vi "Aladdin 2 build.vi"() -> ()   [LabVIEW 2020]
uses:
  <vilib>/Instr/_visa.llb/VISA Configure Serial Port (Instr).vi
panel:
  in  "stop":bool
  in  "Mode":enum32{"Setup", "Run"}(tab)
  out "Min rate 2":dbl caption="Min rate" format="%#_4g"
  in  "Target Volume2":dbl caption="Target Vol (ul)"
  in  "Send 2":bool
  in  "Address2":string(combo) caption="Address"
  in  "Dia (mm)2":dbl=0.1 caption="Dia (mm)" min=0.1 max=50.0
  out "Max rate ml/min2":dbl caption="Max rate" format="%#_4g"
  in  "Direction2":string(combo)="inf" caption="Direction"
  in  "Serial Reset":bool
  in  "Target Vol":dbl caption="Target Vol (ul)"
  in  "Send":bool
  in  "Address":string(combo)
  in  "dia (mm)":dbl=0.1 caption="Dia (mm)" min=0.1 max=50.0
  out "Max rate":dbl format="%#_4g"
  in  "Direction":string(combo)="inf"
  in  "Serial Port":refnum<visa-resource-name>="COM1"
  in  "Pumps":string(combo)="1"
  in  "Set rate":dbl format="%#_4g"
  in  "Flow rate2":dbl caption="Set rate"
  out "Min rate":dbl format="%#_4g"
  in  "Units":string(combo)="mm"
  in  "Units2":string(combo)="mm" caption="Units"
  out "Dispensed 2":string caption="Dispensed"
  out "Dispensed":string
  out "Direction1":string caption="Direction"
  in  "Go 2":bool
  in  "Go 1":bool
  out "Target2":string caption="Target"
  out "Target1":string caption="Target"
  out "Direction2":string caption="Direction"
  out "Rate2":string caption="Rate"
  out "Rate1":string caption="Rate"
  in  "Reset1 2":bool
  in  "Reset1":bool
  # "Pump 1"
  # "Pump 2"
  # "Set pump Baud rate to 19200"
  # "Pump 1"
  # "Pump 2"
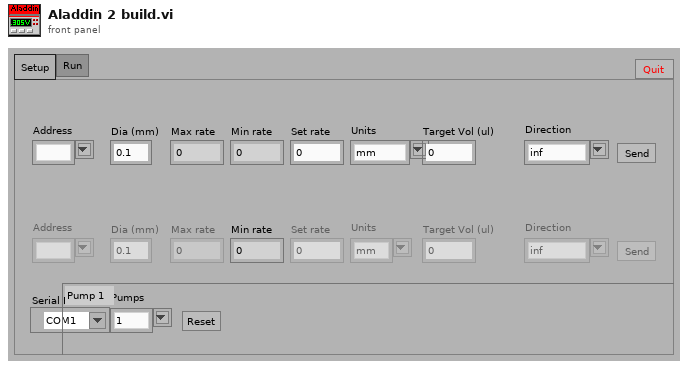
[diagram p1: front panel]
types:
  T1 = enum8{"Enabled", "Disabled", "Disabled and Grayed Out"}
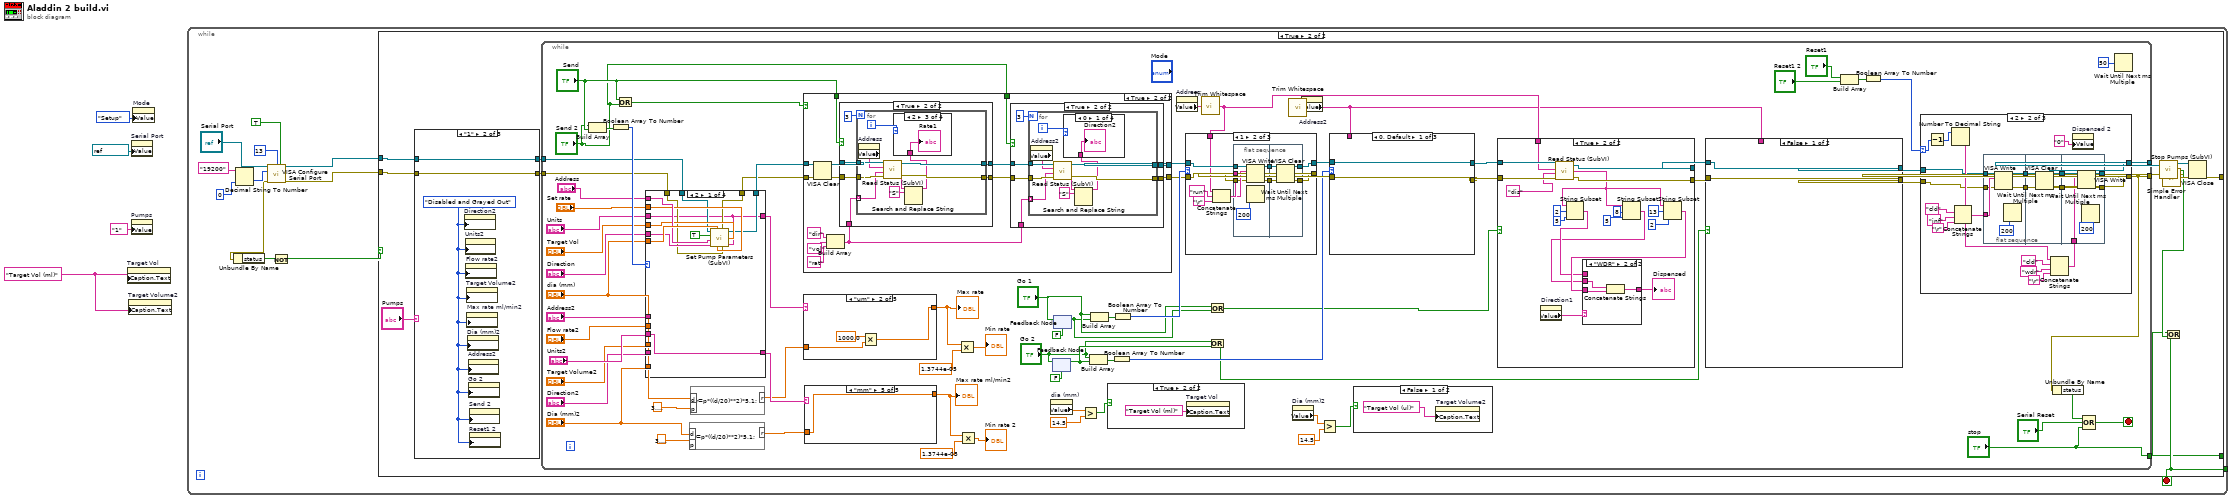
[diagram p0: block diagram]
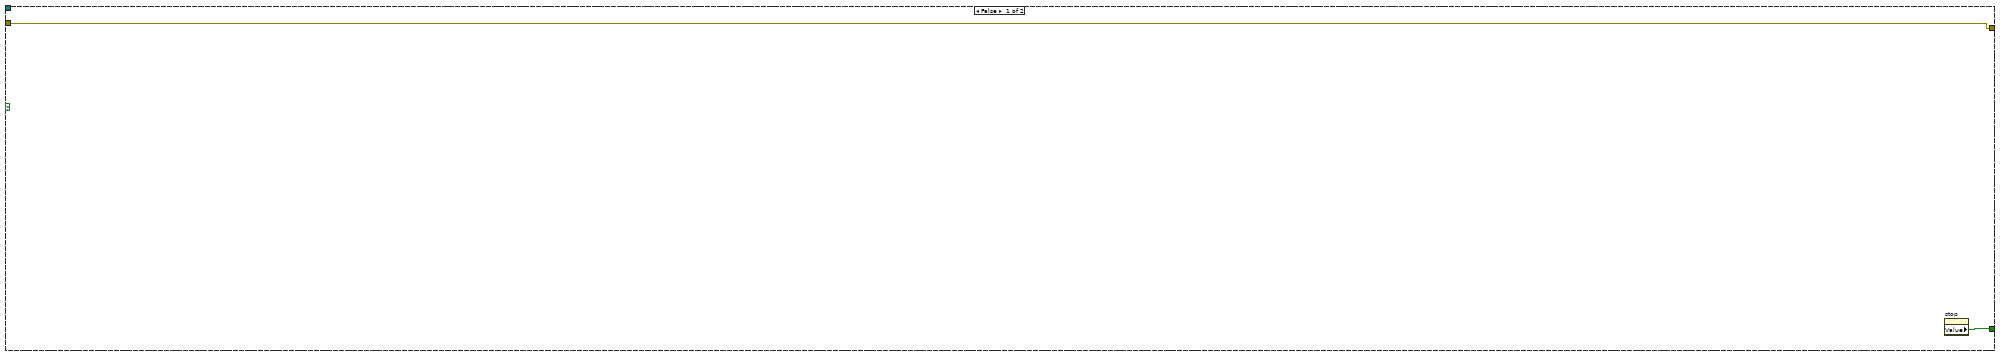
[diagram p2: hidden frame]
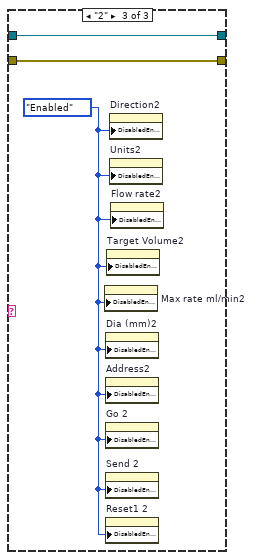
[diagram p4: hidden frame]
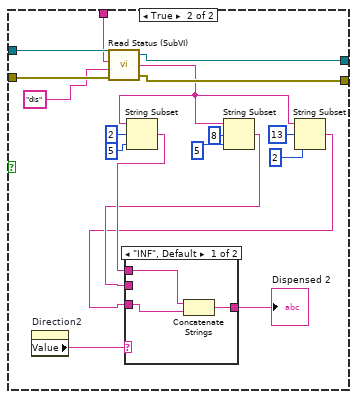
[diagram p5: hidden frame]
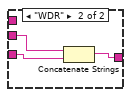
[diagram p6: hidden frame]
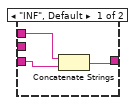
[diagram p8: hidden frame]
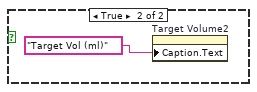
[diagram p9: hidden frame]
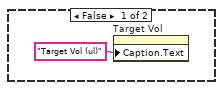
[diagram p10: hidden frame]
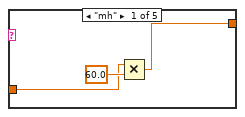
[diagram p11: hidden frame]
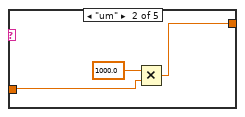
[diagram p12: hidden frame]
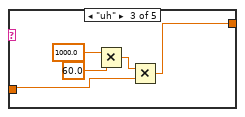
[diagram p13: hidden frame]
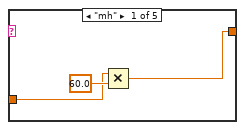
[diagram p15: hidden frame]
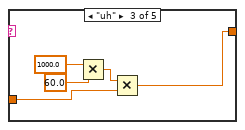
[diagram p16: hidden frame]
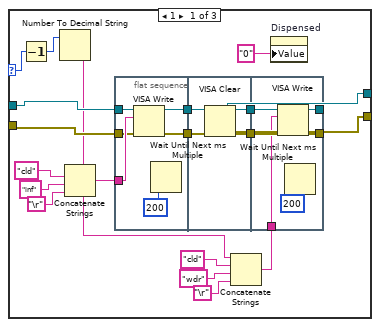
[diagram p19: hidden frame]
diagram:
  w1 = "Target Vol (ml)" ("Caption.Text")
  n1 = property on="Target Vol" class="DigNum (strict)"("Caption.Text"=w1) -> ()  [unwired: 2 in, 2 out]
  n2 = property on="Target Volume2" class="DigNum (strict)"("Caption.Text"=w1) -> ()  [unwired: 2 in, 2 out]
  n3 = property on="Serial Port" class="VISAName"("Value"=refnum<visa-resource-name> "COM1" ("Serial Port")) -> ()  [unwired: 2 in, 2 out]
  n4 = property on="Pumps" class="CmbBox"("Value"="1" ("Pumps")) -> ()  [unwired: 2 in, 2 out]
  n5 = property on="Mode" class="TabCtl (strict)"("Value"=enum32{"Setup", "Run"}."Setup" ("Mode")) -> ()  [unwired: 2 in, 2 out]
  n6 = while {
    tunnel: [w7] -> _
    stop <- w7 stop-if-true
    n7 = Decimal String To Number(string="19200" ("Baud Rate"), default (0L)=u32 0 ("default (0 I32)")) -> (number=w14:u32)  [unwired: 1 in, 1 out]
    n8 = call-poly "VISA Configure Serial Port"("VISA resource name"="Serial Port", "termination char\n(0xA = '\\n' = LF)"=u8 13 ("termination char\n(0xA = '\\n' = LF)"), "Enable Termination\nChar (T)"=TRUE ("Enable Termination\nChar (T)"), "baud rate (9600)"=w14) -> ("VISA resource name out"=w12:refnum<visa-resource-name>, "error out"=w10:errorcluster)  [unwired: 10 in]
    n9 = Unbundle By Name(w10) -> ("status"=w9:bool)
    n10 = Not(x=w9) -> (.not. x?=w8:bool)
    n11 = case shown="True" w8 {
      tunnel: w12 -> [_ w28]
      tunnel: w10 -> [w20 w27]
      tunnel: [w19 w24] -> w5
      tunnel: [w20 w21] -> w11
      frame False {
        n12 = property on="stop" class="Bool (strict)"() -> ("Value"=w19:bool)  [unwired: 2 in, 2 out]
      }
      frame True {
        n13 = case shown="\"1\"" "Pumps" {
          tunnel: w28 -> [w33 w35 w38]
          tunnel: w27 -> [w32 w34 w37]
          tunnel: [w33 w35 w38] -> w26
          tunnel: [w32 w34 w37] -> w25
          frame Default {
          }
          frame "1" {
            w36 = T1."Disabled and Grayed Out" ("Disabled")
            n14 = property on="Direction2" class="CmbBox"("DisabledEnum"=w36) -> ()  [unwired: 2 in, 2 out]
            n15 = property on="Units2" class="CmbBox"("DisabledEnum"=w36) -> ()  [unwired: 2 in, 2 out]
            n16 = property on="Flow rate2" class="DigNum (strict)"("DisabledEnum"=w36) -> ()  [unwired: 2 in, 2 out]
            n17 = property on="Target Volume2" class="DigNum (strict)"("DisabledEnum"=w36) -> ()  [unwired: 2 in, 2 out]
            n18 = property on="Max rate ml/min2" class="DigNum (strict)"("DisabledEnum"=w36) -> ()  [unwired: 2 in, 2 out]
            n19 = property on="Dia (mm)2" class="DigNum (strict)"("DisabledEnum"=w36) -> ()  [unwired: 2 in, 2 out]
            n20 = property on="Address2" class="CmbBox"("DisabledEnum"=w36) -> ()  [unwired: 2 in, 2 out]
            n21 = property on="Go 2" class="Bool (strict)"("DisabledEnum"=w36) -> ()  [unwired: 2 in, 2 out]
            n22 = property on="Send 2" class="Bool"("DisabledEnum"=w36) -> ()  [unwired: 2 in, 2 out]
            n23 = property on="Reset1 2" class="Bool"("DisabledEnum"=w36) -> ()  [unwired: 2 in, 2 out]
          }
          frame "2" {
            w39 = T1."Enabled" ("Disabled")
            n24 = property on="Max rate ml/min2" class="DigNum (strict)"("DisabledEnum"=w39) -> ()  [unwired: 2 in, 2 out]
            n25 = property on="Dia (mm)2" class="DigNum (strict)"("DisabledEnum"=w39) -> ()  [unwired: 2 in, 2 out]
            n26 = property on="Address2" class="CmbBox"("DisabledEnum"=w39) -> ()  [unwired: 2 in, 2 out]
            n27 = property on="Go 2" class="Bool (strict)"("DisabledEnum"=w39) -> ()  [unwired: 2 in, 2 out]
            n28 = property on="Send 2" class="Bool"("DisabledEnum"=w39) -> ()  [unwired: 2 in, 2 out]
            n29 = property on="Reset1 2" class="Bool"("DisabledEnum"=w39) -> ()  [unwired: 2 in, 2 out]
            n30 = property on="Target Volume2" class="DigNum (strict)"("DisabledEnum"=w39) -> ()  [unwired: 2 in, 2 out]
            n31 = property on="Direction2" class="CmbBox"("DisabledEnum"=w39) -> ()  [unwired: 2 in, 2 out]
            n32 = property on="Units2" class="CmbBox"("DisabledEnum"=w39) -> ()  [unwired: 2 in, 2 out]
            n33 = property on="Flow rate2" class="DigNum (strict)"("DisabledEnum"=w39) -> ()  [unwired: 2 in, 2 out]
          }
        }
        n34 = while {
          tunnel: w25 -> [w87]
          tunnel: w26 -> [w88]
          tunnel: ["stop"] -> w24
          tunnel: [w79] -> w30
          tunnel: [w59] -> w29
          stop <- w114 stop-if-true
          n35 = Build Array("Send 2", "Send") -> (w101:bool[])
          n36 = Boolean Array To Number(Boolean array=w101) -> (number=w100:u32)
          n37 = Or(x="Send", y="Send 2") -> (x .or. y?=w89:bool)
          n38 = case shown="2" w100 {
            tunnel: "Address" -> [w281 _ _ _]
            tunnel: "Set rate" -> [w279 _ _ _]
            tunnel: "Units" -> [w273 w286 w297 w301]
            tunnel: "Target Vol" -> [w278 _ _ _]
            tunnel: "Direction" -> [w280 _ _ _]
            tunnel: "dia (mm)" -> [w283 _ _ _]
            tunnel: "Address2" -> [_ w295 _ _]
            tunnel: "Flow rate2" -> [_ w294 _ _]
            tunnel: "Units2" -> [w272 w284 w296 w300]
            tunnel: "Target Volume2" -> [_ w293 _ _]
            tunnel: "Direction2" -> [_ w285 _ _]
            tunnel: "Dia (mm)2" -> [_ w292 _ _]
            tunnel: w88 -> [w275 w290 w298 w304]
            tunnel: w87 -> [w274 w289 w299 w303]
            tunnel: [w276 w288 w298 w304] -> w86
            tunnel: [w277 w287 w299 w303] -> w85
            tunnel: [w273 w286 w297 w301] -> w73
            tunnel: [w272 w284 w296 w300] -> w72
            frame 2 {
              n39 = call "Set Pump Parameters (SubVI).vi"("Units"=w273, "error in"=w274, "Target Volume"=w278, "Flow rate"=w279, "Direction"=w280, "Pump Add"=w281, "diameter (mm)"=w283, "Send"=TRUE, "VISA resource name in"=w275) -> ("VISA resource name out"=w276:refnum<visa-resource-name>, "error out"=w277:errorcluster)
            }
            frame 1 {
              n40 = call "Set Pump Parameters (SubVI).vi"("Units"=w284, "error in"=w289, "Target Volume"=w293, "Flow rate"=w294, "Direction"=w285, "Pump Add"=w295, "diameter (mm)"=w292, "Send"=TRUE, "VISA resource name in"=w290) -> ("VISA resource name out"=w288:refnum<visa-resource-name>, "error out"=w287:errorcluster)
            }
            frame Default {
            }
            frame 3 {
              n41 = call "Set Pump Parameters (SubVI).vi"("Send"=FALSE) -> ()  [unwired: 8 in, 2 out]
            }
          }
          n42 = formula code="r=p*((d/20)**2)*5.1;"("d"="Dia (mm)2", "p"=3.141592653589793) -> ("r"=w70:dbl)
          n43 = formula code="r=p*((d/20)**2)*5.1;"("d"="dia (mm)", "p"=3.141592653589793) -> ("r"=w71:dbl)
          n44 = case shown="True" w89 {
            tunnel: [w390 w394] -> w105
            tunnel: [w389 w393] -> w104
            tunnel: w86 -> [w390 w399]
            tunnel: w85 -> [w389 w398]
            tunnel: "Send" -> [_ w392]
            tunnel: "Send 2" -> [_ w391]
            frame False {
            }
            frame True {
              n45 = VISA Clear(VISA resource name=w399, error in (no error)=w398) -> (VISA resource name out=w401:refnum<visa-resource-name>, error out=w400:errorcluster)
              n46 = Build Array("dir", "vol", "rat") -> (w395:string[])
              n47 = case shown="True" w392 {
                tunnel: [w427 w433] -> w397
                tunnel: [w426 w432] -> w396
                tunnel: w395 -> [_ w431]
                tunnel: w401 -> [w427 w430]
                tunnel: w400 -> [w426 w429]
                frame False {
                }
                frame True {
                  n48 = for {
                    N: 3 -> [_]
                    tunnel: w430 -> [w443]
                    tunnel: w429 -> [w442]
                    tunnel: w431 -> [w441] mode=indexing
                    tunnel: [w440] -> w433
                    tunnel: [w439] -> w432
                    i -> [w435]
                    n49 = property on="Address" class="CmbBox"() -> ("Value"=w434:string)  [unwired: 2 in, 2 out]
                    n50 = call "Read Status (SubVI).vi"("error out 2"=w442, "String"=w441, "String 2"=w434, "VISA resource name out 2"=w443) -> ("error out"=w439:errorcluster, "read buffer"=w437:string, "VISA resource name out"=w440:refnum<visa-resource-name>)
                    n51 = Search and Replace String(input string=w437, search string="S") -> (result string=w436:string)  [unwired: 6 in, 3 out]
                    n52 = case shown="2" w435 {
                      tunnel: w436 -> [w444 w445 w446 _]
                      frame 0 {
                        "Direction1" <- w444
                      }
                      frame 1 {
                        "Target1" <- w445
                      }
                      frame 2 {
                        "Rate1" <- w446
                      }
                      frame Default {
                      }
                    }
                  }
                }
              }
              n53 = case shown="True" w391 {
                tunnel: [w406 w412] -> w394
                tunnel: [w405 w411] -> w393
                tunnel: w395 -> [_ w410]
                tunnel: w397 -> [w406 w409]
                tunnel: w396 -> [w405 w408]
                frame False {
                }
                frame True {
                  n54 = for {
                    N: 3 -> [_]
                    tunnel: w409 -> [w422]
                    tunnel: w408 -> [w421]
                    tunnel: w410 -> [w420] mode=indexing
                    tunnel: [w419] -> w412
                    tunnel: [w418] -> w411
                    i -> [w414]
                    n55 = property on="Address2" class="CmbBox"() -> ("Value"=w413:string)  [unwired: 2 in, 2 out]
                    n56 = call "Read Status (SubVI).vi"("error out 2"=w421, "String"=w420, "String 2"=w413, "VISA resource name out 2"=w422) -> ("error out"=w418:errorcluster, "read buffer"=w416:string, "VISA resource name out"=w419:refnum<visa-resource-name>)
                    n57 = Search and Replace String(input string=w416, search string="S") -> (result string=w415:string)  [unwired: 6 in, 3 out]
                    n58 = case shown="0" w414 {
                      tunnel: w415 -> [w423 w424 w425 _]
                      frame 0 {
                        "Direction2" <- w423
                      }
                      frame 1 {
                        "Target2" <- w424
                      }
                      frame 2 {
                        "Rate2" <- w425
                      }
                      frame Default {
                      }
                    }
                  }
                }
              }
            }
          }
          n59 = case shown="\"um\"" w73 {
            tunnel: w71 -> [w186 w188 w192 w196 w197]
            tunnel: [w185 w189 w191 w196 w197] -> w64
            frame "mh" {
              n60 = Multiply(x=w186, y=60.0) -> (x*y=w185:dbl)
            }
            frame "um" {
              n61 = Multiply(x=1000.0, y=w188) -> (x*y=w189:dbl)
            }
            frame "uh" {
              n62 = Multiply(x=1000.0, y=60.0) -> (x*y=w195:dbl)
              n63 = Multiply(x=w195, y=w192) -> (x*y=w191:dbl)
            }
            frame Default {
            }
            frame "mm" {
            }
          }
          "Max rate" <- w64
          n64 = case shown="\"mm\"" w72 {
            tunnel: w70 -> [w172 w176 w179 w183 w184]
            tunnel: [w173 w175 w178 w183 w184] -> w68
            frame "mh" {
              n65 = Multiply(x=w172, y=60.0) -> (x*y=w173:dbl)
            }
            frame "um" {
              n66 = Multiply(x=1000.0, y=w176) -> (x*y=w175:dbl)
            }
            frame "uh" {
              n67 = Multiply(x=1000.0, y=60.0) -> (x*y=w180:dbl)
              n68 = Multiply(x=w180, y=w179) -> (x*y=w178:dbl)
            }
            frame Default {
            }
            frame "mm" {
            }
          }
          "Max rate ml/min2" <- w68
          n69 = Multiply(x=w64, y=1.3744e-05) -> (x*y=→"Min rate":dbl)
          n70 = Multiply(x=w68, y=1.3744e-05) -> (x*y=→"Min rate 2":dbl)
          n71 = property on="dia (mm)" class="DigNum (strict)"() -> ("Value"=w63:dbl)  [unwired: 2 in, 2 out]
          n72 = feedback-in #1("Go 2") -> ()
          n73 = feedback #1(FALSE ("Go 1")) -> (w47:bool)
          n74 = feedback-in #2("Go 1") -> ()
          n75 = feedback #2(FALSE ("Go 1")) -> (w48:bool)
          n76 = Greater?(x=w63, y=14.5) -> (0:w61:bool)
          n77 = Build Array("Go 2", w47) -> (w109:bool[])
          n78 = Build Array("Go 1", w48) -> (w110:bool[])
          n79 = case shown="True" w61 {
            frame False {
              n80 = property on="Target Vol" class="DigNum (strict)"("Caption.Text"="Target Vol (ul)") -> ()  [unwired: 2 in, 2 out]
            }
            frame True {
              n81 = property on="Target Vol" class="DigNum (strict)"("Caption.Text"="Target Vol (ml)") -> ()  [unwired: 2 in, 2 out]
            }
          }
          n82 = Boolean Array To Number(Boolean array=w109) -> (number=w54:u32)
          n83 = Boolean Array To Number(Boolean array=w110) -> (number=w111:u32)
          n84 = property on="Address" class="CmbBox"() -> ("Value"=w53:string)  [unwired: 2 in, 2 out]
          n85 = call <vilib>:"Trim Whitespace.vi"("string"=w53) -> ("trimmed string"=w43:string)  [unwired: 1 in]
          n86 = case shown="1" w111 {
            tunnel: [w348 w351 w375] -> w107
            tunnel: [w347 w350 w374] -> w106
            tunnel: w105 -> [w348 w355 w373]
            tunnel: w104 -> [w347 w354 w372]
            tunnel: w43 -> [_ w349 w369]
            frame 0, Default {
            }
            frame 1 {
              n87 = Concatenate Strings(w349, "run" ("string"), "\r") -> (w356:string)
              n88 = flat-sequence {
                tunnel: w356 -> [w364]
                tunnel: w355 -> [w363]
                tunnel: w354 -> [w362]
                tunnel: [w361] -> w353
                tunnel: [w360] -> w352
                tunnel: w353 -> [w368]
                tunnel: w352 -> [w367]
                tunnel: [w366] -> w351
                tunnel: [w365] -> w350
                frame #0 {
                  n89 = VISA Write(VISA resource name=w363, write buffer=w364, error in (no error)=w362) -> (VISA resource name out=w361:refnum<visa-resource-name>, error out=w360:errorcluster)  [unwired: 1 out]
                  n90 = Wait Until Next ms Multiple(millisecond multiple=u32 200) -> ()  [unwired: 1 out]
                }
                frame #1 {
                  n91 = VISA Clear(VISA resource name=w368, error in (no error)=w367) -> (VISA resource name out=w366:refnum<visa-resource-name>, error out=w365:errorcluster)
                }
              }
            }
            frame 2 {
              n92 = Concatenate Strings(w369, "stp" ("string"), "\r") -> (w376:string)
              n93 = flat-sequence {
                tunnel: w376 -> [w384]
                tunnel: w373 -> [w381]
                tunnel: w372 -> [w380]
                tunnel: [w383] -> w371
                tunnel: [w382] -> w370
                tunnel: [w388] -> w374
                tunnel: [w385] -> w375
                tunnel: w371 -> [w387]
                tunnel: w370 -> [w386]
                frame #0 {
                  n94 = Wait Until Next ms Multiple(millisecond multiple=u32 200) -> ()  [unwired: 1 out]
                  n95 = VISA Write(VISA resource name=w381, write buffer=w384, error in (no error)=w380) -> (VISA resource name out=w383:refnum<visa-resource-name>, error out=w382:errorcluster)  [unwired: 1 out]
                }
                frame #1 {
                  n96 = VISA Clear(VISA resource name=w387, error in (no error)=w386) -> (VISA resource name out=w385:refnum<visa-resource-name>, error out=w388:errorcluster)
                }
              }
            }
          }
          n97 = Or(x="Go 2", y=w47) -> (x .or. y?=w44:bool)
          n98 = Or(x="Go 1", y=w48) -> (x .or. y?=w45:bool)
          n99 = property on="Dia (mm)2" class="DigNum (strict)"() -> ("Value"=w56:dbl)  [unwired: 2 in, 2 out]
          n100 = property on="Address2" class="CmbBox"() -> ("Value"=w52:string)  [unwired: 2 in, 2 out]
          n101 = call <vilib>:"Trim Whitespace.vi"("string"=w52) -> ("trimmed string"=w42:string)  [unwired: 1 in]
          n102 = Greater?(x=w56, y=14.5) -> (0:w55:bool)
          n103 = case shown="0, Default" w54 {
            tunnel: w107 -> [w306 w313 w333]
            tunnel: w106 -> [w305 w312 w332]
            tunnel: [w306 w311 w331] -> w103
            tunnel: [w305 w310 w330] -> w102
            tunnel: w42 -> [_ w307 w327]
            frame 0, Default {
            }
            frame 1 {
              n104 = Concatenate Strings(w307, "run" ("string"), "\r") -> (w314:string)
              n105 = flat-sequence {
                tunnel: w314 -> [w322]
                tunnel: w313 -> [w321]
                tunnel: w312 -> [w320]
                tunnel: [w319] -> w309
                tunnel: [w318] -> w308
                tunnel: [w323] -> w310
                tunnel: [w324] -> w311
                tunnel: w309 -> [w325]
                tunnel: w308 -> [w326]
                frame #0 {
                  n106 = VISA Write(VISA resource name=w321, write buffer=w322, error in (no error)=w320) -> (VISA resource name out=w319:refnum<visa-resource-name>, error out=w318:errorcluster)  [unwired: 1 out]
                  n107 = Wait Until Next ms Multiple(millisecond multiple=u32 200) -> ()  [unwired: 1 out]
                }
                frame #1 {
                  n108 = VISA Clear(VISA resource name=w325, error in (no error)=w326) -> (VISA resource name out=w324:refnum<visa-resource-name>, error out=w323:errorcluster)
                }
              }
            }
            frame 2 {
              n109 = Concatenate Strings(w327, "stp" ("string"), "\r") -> (w334:string)
              n110 = flat-sequence {
                tunnel: w334 -> [w342]
                tunnel: w333 -> [w341]
                tunnel: w332 -> [w340]
                tunnel: [w339] -> w329
                tunnel: [w338] -> w328
                tunnel: [w343] -> w330
                tunnel: [w344] -> w331
                tunnel: w329 -> [w345]
                tunnel: w328 -> [w346]
                frame #0 {
                  n111 = VISA Write(VISA resource name=w341, write buffer=w342, error in (no error)=w340) -> (VISA resource name out=w339:refnum<visa-resource-name>, error out=w338:errorcluster)  [unwired: 1 out]
                  n112 = Wait Until Next ms Multiple(millisecond multiple=u32 200) -> ()  [unwired: 1 out]
                }
                frame #1 {
                  n113 = VISA Clear(VISA resource name=w345, error in (no error)=w346) -> (VISA resource name out=w344:refnum<visa-resource-name>, error out=w343:errorcluster)
                }
              }
            }
          }
          n114 = case shown="False" w55 {
            frame False {
              n115 = property on="Target Volume2" class="DigNum (strict)"("Caption.Text"="Target Vol (ul)") -> ()  [unwired: 2 in, 2 out]
            }
            frame True {
              n116 = property on="Target Volume2" class="DigNum (strict)"("Caption.Text"="Target Vol (ml)") -> ()  [unwired: 2 in, 2 out]
            }
          }
          n117 = case shown="True" w45 {
            tunnel: [w143 w161] -> w51
            tunnel: [w142 w160] -> w50
            tunnel: w103 -> [w143 w159]
            tunnel: w102 -> [w142 w158]
            tunnel: w43 -> [_ w149]
            frame False {
            }
            frame True {
              n118 = property on="Direction1" class="Str"() -> ("Value"=w148:string)  [unwired: 2 in, 2 out]
              n119 = call "Read Status (SubVI).vi"("error out 2"=w158, "String"="dis" ("string"), "String 2"=w149, "VISA resource name out 2"=w159) -> ("error out"=w160:errorcluster, "read buffer"=w155:string, "VISA resource name out"=w161:refnum<visa-resource-name>)
              n120 = String Subset(string=w155, offset (0)=2, length (rest)=5 ("length (rest)")) -> (substring=w145:string)
              n121 = String Subset(string=w155, offset (0)=8, length (rest)=5 ("length (rest)")) -> (substring=w144:string)
              n122 = String Subset(string=w155, offset (0)=13, length (rest)=2 ("length (rest)")) -> (substring=w146:string)
              n123 = case shown="\"WDR\"" w148 {
                tunnel: [w164 w167] -> w147
                tunnel: w146 -> [w163 w165]
                tunnel: w145 -> [w162 _]
                tunnel: w144 -> [_ w166]
                frame "INF", Default {
                  n124 = Concatenate Strings(w162, w163) -> (w164:string)
                }
                frame "WDR" {
                  n125 = Concatenate Strings(w166, w165) -> (w167:string)
                }
              }
              "Dispensed" <- w147
            }
          }
          n126 = case shown="False" w44 {
            tunnel: [w117 w135] -> w81
            tunnel: [w116 w134] -> w80
            tunnel: w51 -> [w117 w133]
            tunnel: w50 -> [w116 w132]
            tunnel: w42 -> [_ w123]
            frame False {
            }
            frame True {
              n127 = property on="Direction2" class="Str"() -> ("Value"=w122:string)  [unwired: 2 in, 2 out]
              n128 = call "Read Status (SubVI).vi"("error out 2"=w132, "String"="dis" ("string"), "String 2"=w123, "VISA resource name out 2"=w133) -> ("error out"=w134:errorcluster, "read buffer"=w129:string, "VISA resource name out"=w135:refnum<visa-resource-name>)
              n129 = String Subset(string=w129, offset (0)=2, length (rest)=5 ("length (rest)")) -> (substring=w120:string)
              n130 = String Subset(string=w129, offset (0)=8, length (rest)=5 ("length (rest)")) -> (substring=w119:string)
              n131 = String Subset(string=w129, offset (0)=13, length (rest)=2 ("length (rest)")) -> (substring=w118:string)
              n132 = case shown="\"INF\", Default" w122 {
                tunnel: [w138 w141] -> w121
                tunnel: w120 -> [w136 _]
                tunnel: w119 -> [_ w139]
                tunnel: w118 -> [w137 w140]
                frame "INF", Default {
                  n133 = Concatenate Strings(w136, w137) -> (w138:string)
                }
                frame "WDR" {
                  n134 = Concatenate Strings(w139, w140) -> (w141:string)
                }
              }
              "Dispensed 2" <- w121
            }
          }
          n135 = Build Array("Reset1", "Reset1 2") -> (w76:bool[])
          n136 = Boolean Array To Number(Boolean array=w76) -> (number=w74:u32)
          n137 = case shown="2" w74 {
            selector: w74 -> [w198 w239 _]
            tunnel: w81 -> [w213 w238 w271]
            tunnel: w80 -> [w212 w237 w270]
            tunnel: [w211 w236 w271] -> w79
            tunnel: [w210 w235 w270] -> w59
            frame 1 {
              n138 = Decrement(x=w198) -> (x-1=w199:u32)
              n139 = Number To Decimal String(number=w199) -> (decimal integer string=w200:string)  [unwired: 1 in]
              n140 = Concatenate Strings(w200, "cld" ("string"), "inf" ("string"), "\r") -> (w214:string)
              n141 = flat-sequence {
                tunnel: w214 -> [w223]
                tunnel: w213 -> [w222]
                tunnel: w212 -> [w221]
                tunnel: [w220] -> w217
                tunnel: [w219] -> w216
                tunnel: w217 -> [w226]
                tunnel: w216 -> [w227]
                tunnel: [w225] -> w206
                tunnel: [w224] -> w205
                tunnel: [w230] -> w210
                tunnel: [w231] -> w211
                tunnel: w206 -> [w232]
                tunnel: w205 -> [w233]
                tunnel: w201 -> [w228]
                frame #0 {
                  n142 = VISA Write(VISA resource name=w222, write buffer=w223, error in (no error)=w221) -> (VISA resource name out=w220:refnum<visa-resource-name>, error out=w219:errorcluster)  [unwired: 1 out]
                  n143 = Wait Until Next ms Multiple(millisecond multiple=u32 200) -> ()  [unwired: 1 out]
                }
                frame #1 {
                  n144 = VISA Clear(VISA resource name=w226, error in (no error)=w227) -> (VISA resource name out=w225:refnum<visa-resource-name>, error out=w224:errorcluster)
                }
                frame #2 {
                  n145 = VISA Write(VISA resource name=w232, write buffer=w228, error in (no error)=w233) -> (VISA resource name out=w231:refnum<visa-resource-name>, error out=w230:errorcluster)  [unwired: 1 out]
                  n146 = Wait Until Next ms Multiple(millisecond multiple=u32 200) -> ()  [unwired: 1 out]
                }
              }
              n147 = Concatenate Strings(w200, "cld" ("string"), "wdr" ("string"), "\r") -> (w201:string)
              n148 = property on="Dispensed" class="Str"("Value"="0" ("Vol Infused")) -> ()  [unwired: 2 in, 2 out]
            }
            frame 2 {
              n149 = Decrement(x=w239) -> (x-1=w240:u32)
              n150 = Number To Decimal String(number=w240) -> (decimal integer string=w241:string)  [unwired: 1 in]
              n151 = Concatenate Strings(w241, "cld" ("string"), "inf" ("string"), "\r") -> (w248:string)
              n152 = flat-sequence {
                tunnel: w248 -> [w259]
                tunnel: w238 -> [w258]
                tunnel: w237 -> [w257]
                tunnel: [w256] -> w253
                tunnel: [w255] -> w252
                tunnel: w253 -> [w262]
                tunnel: w252 -> [w263]
                tunnel: [w261] -> w251
                tunnel: [w260] -> w250
                tunnel: [w266] -> w235
                tunnel: [w267] -> w236
                tunnel: w251 -> [w268]
                tunnel: w250 -> [w269]
                tunnel: w242 -> [w264]
                frame #0 {
                  n153 = VISA Write(VISA resource name=w258, write buffer=w259, error in (no error)=w257) -> (VISA resource name out=w256:refnum<visa-resource-name>, error out=w255:errorcluster)  [unwired: 1 out]
                  n154 = Wait Until Next ms Multiple(millisecond multiple=u32 200) -> ()  [unwired: 1 out]
                }
                frame #1 {
                  n155 = VISA Clear(VISA resource name=w262, error in (no error)=w263) -> (VISA resource name out=w261:refnum<visa-resource-name>, error out=w260:errorcluster)
                }
                frame #2 {
                  n156 = VISA Write(VISA resource name=w268, write buffer=w264, error in (no error)=w269) -> (VISA resource name out=w267:refnum<visa-resource-name>, error out=w266:errorcluster)  [unwired: 1 out]
                  n157 = Wait Until Next ms Multiple(millisecond multiple=u32 200) -> ()  [unwired: 1 out]
                }
              }
              n158 = Concatenate Strings(w241, "cld" ("string"), "wdr" ("string"), "\r") -> (w242:string)
              n159 = property on="Dispensed 2" class="Str"("Value"="0" ("Vol Infused")) -> ()  [unwired: 2 in, 2 out]
            }
            frame Default {
            }
          }
          n160 = Unbundle By Name(w59) -> ("status"=w58:bool)
          n161 = Compound Arithmetic op=OR(w58, "Serial Reset", "stop") -> (w114:bool)
          n162 = Wait Until Next ms Multiple(millisecond multiple=u32 50) -> ()  [unwired: 1 out]
        }
        n163 = call "Stop Pumps (SubVI).vi"("error out 2"=w29, "VISA resource name out 2"=w30) -> ("error out"=w22:errorcluster, "VISA resource name out"=w23:refnum<visa-resource-name>)
        n164 = VISA Close(VISA resource name=w23, error in (no error)=w22) -> (error out=w21:errorcluster)
      }
    }
    n165 = call <vilib>:"Simple Error Handler.vi"("error in (no error)"=w11) -> ("error?"=w6:bool)  [unwired: 4 in, 4 out]
    n166 = Or(x=w5, y=w6) -> (x .or. y?=w7:bool)
  }
